vi "X sensor convert meter to V.vi"() -> ()   [LabVIEW 2013]
doc: "This VI convert the X piezo from um to Voltage."
uses:
  Cypher XY LVDT Parameters.vi
panel:
  in  "X coordinate":dbl format="%#_6p"
  out "Sensor X Voltage":dbl
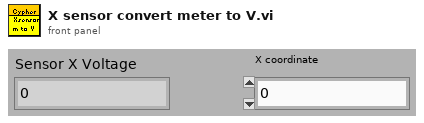
[diagram p1: front panel]
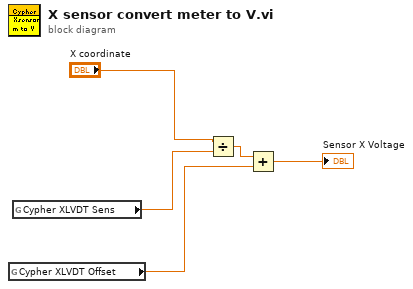
[diagram p0: block diagram]
diagram:
  n1 = global read "Cypher XY LVDT Parameters.vi" "Cypher XLVDT Offset"() -> (w2:dbl)
  n2 = global read "Cypher XY LVDT Parameters.vi" "Cypher XLVDT Sens"() -> (w4:dbl)
  n3 = Divide(x="X coordinate", y=w4) -> (x/y=w3:dbl)
  n4 = Add(x=w3, y=w2) -> (x+y=→"Sensor X Voltage":dbl)
